vi "_PI Send String.vi"(0 "System no.":i32=1 min=1 max=20 step=1, 2 "String to send":string, 3 "Attach termination char.?":bool=TRUE, 5 "error in":errorcluster) -> (19 "error out":errorcluster)   [LabVIEW 2014]
doc: "Sends command with or without trailing termination character to selected system. \n\nValid for all systems."
uses:
  _Available interfaces.ctl
  Public/PI/Mercury/GCS_LabVIEW/Low Level/Communication.llb/Available DLLs.ctl
  _Available DLL interfaces.ctl
  Public/PI/Mercury/GCS_LabVIEW/Low Level/Communication.llb/Termination character.ctl
  Public/PI/Mercury/GCS_LabVIEW/Low Level/Communication.llb/Global1.vi
panel:
  out "Logging mode":bool
  out "Syntax":enum16{"GCS 1.0", "GCS 2.0"}(ring)
  out "Termination character":T1
  out "VISA resource name":refnum<visa-resource-name>
  out "TCP/IP\nConfiguration":T2={"Host address/name"="localhost", "Port"=0, "Board"=4}
  out "DLL Interface Configuration":T5={"DLL for Device"=1, "DLL Interface"=0, "Parameter"=""} {"DLL Interface" items=["RS232", "GPIB", "Board", "TCP-IP", "USB", "RS232_DC"]; "DLL for Device" items=["C-843", "C-844", "E-710", "C-843.PM", "C-865", "E-761", "Mercury", "E-755", "E-753", "C-866", "E-712", "E-725", "E-861", "C-867", "E-517", "E-816"]}
  out "Interface configuration":T7={"RS232 Portnumber"=0, "Timeout"=5000, "RS232 baud rate"=57600, "Interface"=0, "GPIB Bus"=0, "GPIB address"=4, "GPIB Mode"=0} {"Interface" items=["RS232", "GPIB", "DLL", "TCP-IP", "USB", "Analog"]; "RS232 Portnumber" items=["COM1", "COM2", "COM3", "COM4", "COM5", "COM6", "COM7", "COM8", "COM9", "COM10", "COM11", "COM12", "COM13", "COM14", "COM15", "COM16", "COM17", "COM18", "COM19", "COM20", "COM21", "COM22", "COM23", "COM24", "COM25", "COM26", "COM27", "COM28", "COM29", "COM30"]}
  # "This vi sends a string w/o termination character via the selected interface."
  # "Communication setup indicators (for troubleshooting):"
  # "TCP/IP:"
  # "DLL:"
  # "General:"
  # "RS232:"
  # "GPIB:"
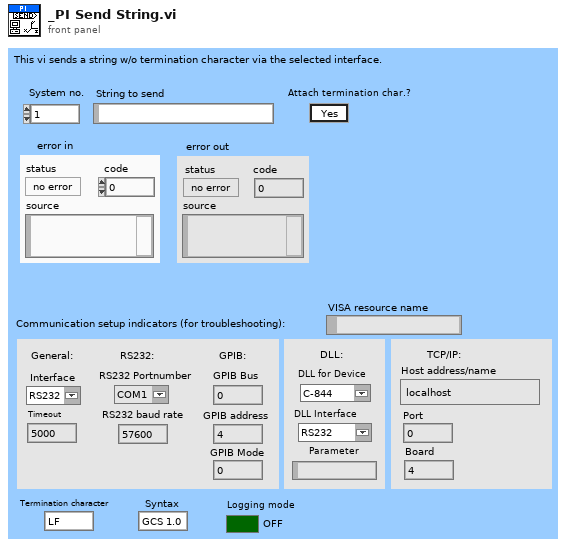
[diagram p1: front panel]
types:
  T1 = typedef "Termination character.ctl" = enum16{"LF", "CR", "LFCR", "CRLF"}
  T2 = cluster{"Host address/name":string, "Port":i32, "Board":i32}
  T3 = typedef "Available DLLs.ctl" = u16
  T4 = typedef "_Available DLL interfaces.ctl" = u16
  T5 = cluster{"DLL for Device":T3, "DLL Interface":T4, "Parameter":string}
  T6 = typedef "_Available interfaces.ctl" = u16
  T7 = cluster{"RS232 Portnumber":u16, "Timeout":u32, "RS232 baud rate":u32, "Interface":T6, "GPIB Bus":i16, "GPIB address":i16, "GPIB Mode":i16}
  T8 = cluster{"Host address/name":string, "Port":i32, "Board":i32}[]
  T9 = typedef "Available interfaces.ctl" = u16
  T10 = cluster{"RS232 Portnumber":i32, "Timeout":i32, "RS232 Baud rate":u32, "Interface":T9, "GPIB Bus":i32, "GPIB Address":i32, "GPIB Mode":i32}[]
  T11 = cluster{"RS232 Portnumber":i32, "Timeout":i32, "RS232 Baud rate":u32, "Interface":T9, "GPIB Bus":i32, "GPIB Address":i32, "GPIB Mode":i32}
  T12 = typedef "Available DLL interfaces.ctl" = u16
  T13 = cluster{"DLL for Device":T3, "DLL Interface":T12, "Parameter":string}[]
  T14 = enum16{"C844_IsDLLAvailable", "C844_ConnectRS232", "C844_ConnectNIgpib", "C844_IsConnected", "C844_CloseConnection", "C844_GcsCommandset", "C844_GetError", "C844_GcsGetAnswerSize", "C844_GcsGetAnswer", "C843_IsDLLAvailable", "C843_Connect", "C843_IsConnected", "C843_CloseConnection", "C843_GcsCommandset", "C843_GetError", "C843_GcsGetAnswerSize", "C843_GcsGetAnswer", "E710_IsDLLAvailable", "E710_ConnectRS232", "E710_ConnectNIgpib", "E710_IsConnected", "E710_CloseConnection", "E710_GcsCommandset", "E710_GetError", "E710_GcsGetAnswerSize", "E710_GcsGetAnswer", "C843_PM_IsDLLAvailable", "C843_PM_Connect", "C843_PM_IsConnected", "C843_PM_CloseConnection", "C843_PM_GcsCommandset", "C843_PM_GetError", "C843_PM_GcsGetAnswerSize", "C843_PM_GcsGetAnswer", "C843_PM_GetCurrentBoardID", "C843_GetCurrentBoardID", "C865_IsDLLAvailable", "C865_ConnectRS232", "C865_IsConnected", "C865_CloseConnection", "C865_GcsCommandset", "C865_GetError", "C865_GcsGetAnswerSize", "C865_GcsGetAnswer", "C865_GetCurrentInterfaceID", "E761_ConnectPciBoard", "DefineSystem", "CloseConnection", "IsConnected", "ConnectRS232", "ConnectNIgpib", "ConnectPciBoard", "ConnectTCPIP", "GetError", "GcsCommandset", "GCSGetAnswerSize", "GcsGetAnswer"}
  T15 = cluster{bool, "DLL I32 Return value":i32, string}
  T16 = cluster{"DLL for Device":T3, "DLL Interface":T12, "Parameter":string}
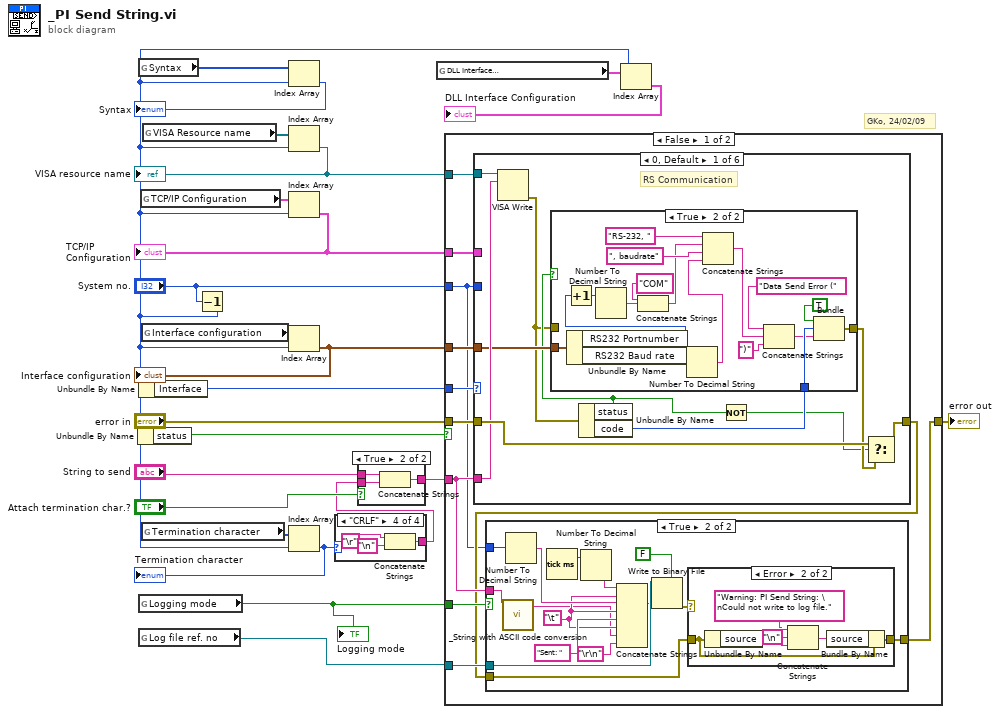
[diagram p0: block diagram]
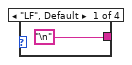
[diagram p2: hidden frame]
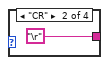
[diagram p3: hidden frame]
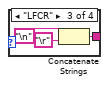
[diagram p4: hidden frame]
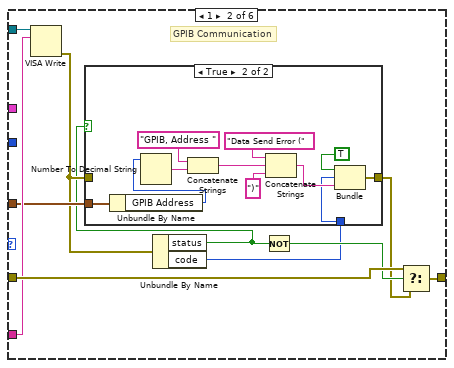
[diagram p9: hidden frame]
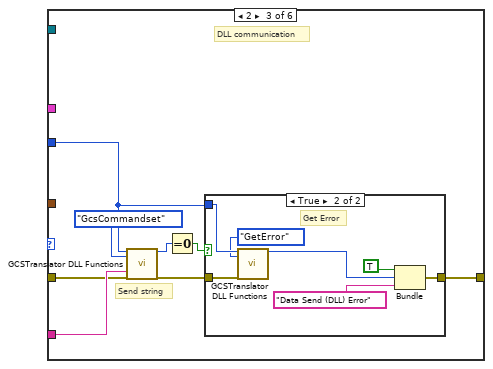
[diagram p11: hidden frame]
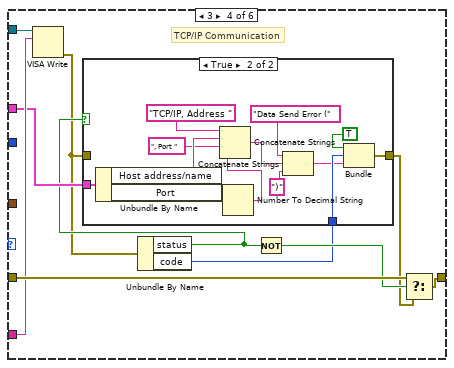
[diagram p13: hidden frame]
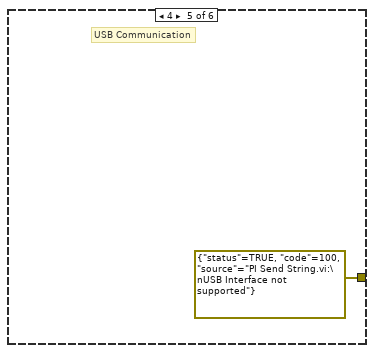
[diagram p15: hidden frame]
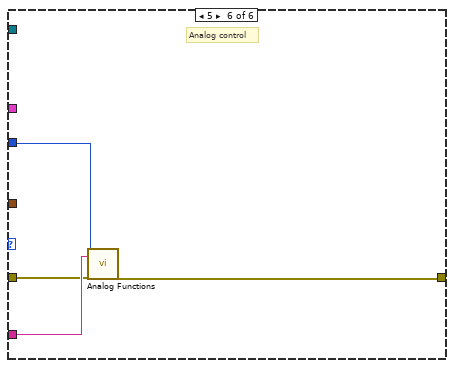
[diagram p16: hidden frame]
diagram:
  # "GKo, 24/02/09"
  n1 = Unbundle By Name("error in") -> ("status"=w24:bool)
  n2 = global read "Global1.vi" "Syntax"() -> (w6:enum16{"GCS 1.0", "GCS 2.0"}[])
  n3 = global read "Global1.vi" "Logging mode"() -> (w1:bool)
  "Logging mode" <- w1
  n4 = global read "Global1.vi" "Log file ref. no"() -> (w2:refnum<file>)
  n5 = global read "Global1.vi" "TCP/IP Configuration"() -> (w12:T8)
  n6 = global read "Global1.vi" "Interface configuration"() -> (w17:T10)
  n7 = global read "Global1.vi" "Termination character"() -> (w7:T1[])
  n8 = global read "Global1.vi" "VISA Resource name"() -> (w11:refnum<visa-resource-name>[])
  n9 = Decrement(x="System no.") -> (x-1=w3:i32)
  n10 = Index Array(array=w6, index=w3) -> (element=→"Syntax":enum16{"GCS 1.0", "GCS 2.0"})
  n11 = Index Array(array=w11, index=w3) -> (element=w10:refnum<visa-resource-name>)
  "VISA resource name" <- w10
  n12 = Index Array(array=w12, index=w3) -> (element=w9:T2)
  "TCP/IP\nConfiguration" <- w9
  n13 = Index Array(array=w17, index=w3) -> (element=w16:T11)
  "Interface configuration" <- w16
  n14 = Unbundle By Name(w16) -> ("Interface"=w18:T9)
  n15 = Index Array(array=w7, index=w3) -> (element=w4:T1)
  "Termination character" <- w4
  n16 = case shown="\"CRLF\"" w4 {
    tunnel: ["\n" "\r" w27 w32] -> w8
    frame "LF", Default {
    }
    frame "CR" {
    }
    frame "LFCR" {
      n17 = Concatenate Strings("\n", "\r") -> (w27:string)
    }
    frame "CRLF" {
      n18 = Concatenate Strings("\r", "\n") -> (w32:string)
    }
  }
  n19 = case shown="True" "Attach termination char.?" {
    tunnel: [w33 w36] -> w20
    tunnel: "String to send" -> [w33 w35]
    tunnel: w8 -> [_ w34]
    frame False {
    }
    frame True {
      n20 = Concatenate Strings(w35, w34) -> (w36:string)
    }
  }
  n21 = global read "Global1.vi" "DLL Interface\nConfiguration"() -> (w15:T13)
  n22 = case shown="False" w24 {
    tunnel: [w38 w166] -> w22
    tunnel: "error in" -> [w47 w166]
    tunnel: w18 -> [w46 _]
    tunnel: w20 -> [w41 _]
    tunnel: w16 -> [w45 _]
    tunnel: "System no." -> [w37 _]
    tunnel: w10 -> [w44 _]
    tunnel: w9 -> [w43 _]
    tunnel: w2 -> [w42 _]
    tunnel: w1 -> [w40 _]
    frame False {
      n23 = case shown="0, Default" w46 {
        tunnel: w47 -> [w80 w108 w126 w146 _ w164]
        tunnel: [w79 w107 w127 w145 errorcluster {"status"=TRUE, "code"=100, "source"="PI Send String.vi:\nUSB Interface not supported"} ("error out") w162] -> w39
        tunnel: w41 -> [w77 w106 w128 w144 _ w165]
        tunnel: w45 -> [w73 w103 _ _ _ _]
        tunnel: w37 -> [_ _ w125 _ _ w163]
        tunnel: w44 -> [w74 w104 _ w142 _ _]
        tunnel: w43 -> [_ _ _ w140 _ _]
        frame 0, Default {
          # "RS Communication"
          n24 = VISA Write(VISA resource name=w74, write buffer=w77) -> (error out=w71:errorcluster)  [unwired: 1 in, 2 out]
          n25 = Unbundle By Name(w71) -> ("status"=w72:bool, "code"=w76:i32)
          n26 = case shown="True" w72 {
            tunnel: [w81 w98] -> w78
            tunnel: w76 -> [_ w96]
            tunnel: w73 -> [_ w88]
            tunnel: w71 -> [w81 _]
            frame False {
            }
            frame True {
              n27 = Unbundle By Name(w88) -> ("RS232 Portnumber"=w83:i32, "RS232 Baud rate"=w87:u32)
              n28 = Increment(x=w83) -> (x+1=w84:i32)
              n29 = Number To Decimal String(number=w84) -> (decimal integer string=w85:string)  [unwired: 1 in]
              n30 = Concatenate Strings("COM" ("string"), w85) -> (w82:string)
              n31 = Number To Decimal String(number=w87) -> (decimal integer string=w91:string)  [unwired: 1 in]
              n32 = Concatenate Strings("RS-232, " ("string"), w82, ", baudrate" ("string"), w91) -> (w89:string)
              n33 = Concatenate Strings("Data Send Error (", w89, ")" ("string")) -> (w95:string)
              n34 = Bundle(TRUE, "code"=w96, w95) -> (w98:cluster{bool, "code":i32, string})  [unwired: 1 in]
            }
          }
          n35 = Not(x=w72) -> (.not. x?=w75:bool)
          n36 = Select(t=w80, s=w75, f=w78) -> (s? t:f=w79:errorcluster)
        }
        frame 1 {
          # "GPIB Communication"
          n37 = VISA Write(VISA resource name=w104, write buffer=w106) -> (error out=w100:errorcluster)  [unwired: 1 in, 2 out]
          n38 = Unbundle By Name(w100) -> ("status"=w99:bool, "code"=w102:i32)
          n39 = case shown="True" w99 {
            tunnel: w103 -> [_ w112]
            tunnel: w102 -> [_ w111]
            tunnel: [w109 w110] -> w101
            tunnel: w100 -> [w109 _]
            frame False {
            }
            frame True {
              n40 = Unbundle By Name(w112) -> ("GPIB Address"=w118:i32)
              n41 = Number To Decimal String(number=w118) -> (decimal integer string=w119:string)  [unwired: 1 in]
              n42 = Concatenate Strings("GPIB, Address " ("string"), w119) -> (w113:string)
              n43 = Concatenate Strings("Data Send Error (", w113, ")" ("string")) -> (w116:string)
              n44 = Bundle(TRUE, "code"=w111, w116) -> (w110:cluster{bool, "code":i32, string})  [unwired: 1 in]
            }
          }
          n45 = Not(x=w99) -> (.not. x?=w105:bool)
          n46 = Select(t=w108, s=w105, f=w101) -> (s? t:f=w107:errorcluster)
        }
        frame 2 {
          # "Send string"
          # "DLL communication"
          n47 = call "GCSTranslator DLL Functions.vi"("System no."=w125, "Function"=T14."GcsCommandset", "String input"=w128, "error in"=w126) -> ("DLL I32 Return value"=w123:i32, "error out"=w122:errorcluster)  [unwired: 11 in, 3 out]
          n48 = Equal To 0?(x=w123) -> (x = 0?=w124:bool)
          n49 = case shown="True" w124 {
            tunnel: [w129 w134] -> w127
            tunnel: w125 -> [_ w131]
            tunnel: w122 -> [w129 w132]
            frame False {
              # "no error"
            }
            frame True {
              # "Get Error"
              n50 = call "GCSTranslator DLL Functions.vi"("System no."=w131, "Function"=T14."GetError", "error in"=w132) -> ("DLL I32 Return value"=w133:i32)  [unwired: 12 in, 4 out]
              n51 = Bundle(TRUE, "DLL I32 Return value"=w133, "Data Send (DLL) Error") -> (w134:T15)  [unwired: 1 in]
            }
          }
        }
        frame 3 {
          # "TCP/IP Communication"
          n52 = VISA Write(VISA resource name=w142, write buffer=w144) -> (error out=w137:errorcluster)  [unwired: 1 in, 2 out]
          n53 = Unbundle By Name(w137) -> ("status"=w138:bool, "code"=w139:i32)
          n54 = case shown="True" w138 {
            tunnel: w137 -> [w147 _]
            tunnel: [w147 w148] -> w141
            tunnel: w140 -> [_ w152]
            tunnel: w139 -> [_ w150]
            frame False {
            }
            frame True {
              n55 = Unbundle By Name(w152) -> ("Host address/name"=w159:string, "Port"=w157:i32)
              n56 = Number To Decimal String(number=w157) -> (decimal integer string=w153:string)  [unwired: 1 in]
              n57 = Concatenate Strings("TCP/IP, Address " ("string"), w159, ", Port " ("string"), w153) -> (w154:string)
              n58 = Concatenate Strings("Data Send Error (", w154, ")" ("string")) -> (w149:string)
              n59 = Bundle(TRUE, "code"=w150, w149) -> (w148:cluster{bool, "code":i32, string})  [unwired: 1 in]
            }
          }
          n60 = Not(x=w138) -> (.not. x?=w143:bool)
          n61 = Select(t=w146, s=w143, f=w141) -> (s? t:f=w145:errorcluster)
        }
        frame 4 {
          # "USB Communication"
        }
        frame 5 {
          # "Analog control"
          n62 = call "Analog Functions.vi"("System no."=w163, "String to send"=w165, "error in"=w164) -> ("error out"=w162:errorcluster)  [unwired: 14 in, 2 out]
        }
      }
      n63 = case shown="True" w40 {
        tunnel: w42 -> [_ w63]
        tunnel: w41 -> [_ w58]
        tunnel: w39 -> [w48 w60]
        tunnel: [w48 w59] -> w38
        tunnel: w37 -> [_ w57]
        frame False {
        }
        frame True {
          w52 = "\t"
          n64 = call "_String with ASCII code conversion.vi"("Input string"=w58) -> ("Output string"=w51:string)  [unwired: 18 in]
          n65 = Number To Decimal String(number=w57) -> (decimal integer string=w54:string)  [unwired: 1 in]
          n66 = Tick Count (ms)() -> (millisecond timer value=w56:u32)
          n67 = Number To Decimal String(number=w56) -> (decimal integer string=w55:string)  [unwired: 1 in]
          n68 = Concatenate Strings(w55, w52, w54, w52, "Sent: " ("string"), w52, w51, "\r\n") -> (w62:string)
          n69 = Write to Binary File(file (use dialog)=w63, data=w62, 5:FALSE ("prepend array or string size? (T)")) -> (error out=w61:errorcluster)  [unwired: 3 in, 2 out]
          n70 = case shown="Error" w61 {
            tunnel: w60 -> [w64 w70]
            tunnel: [w64 w66] -> w59
            frame No Error {
            }
            frame Error {
              n71 = Unbundle By Name(w70) -> ("source"=w69:string)
              n72 = Concatenate Strings(w69, "\n" ("string"), "Warning: PI Send String: \nCould not write to log file." ("source")) -> (w65:string)
              n73 = Bundle By Name(cluster=w70, "source"=w65) -> (w66:errorcluster)
            }
          }
        }
      }
    }
    frame True {
      # "Error!"
    }
  }
  "error out" <- w22
  n74 = Index Array(array=w15, index=w3) -> (element=→"DLL Interface Configuration":T16)
